vi "Divide Quaternion by Scalar.vi"(1 "y":dbl, 2 "quaternion":T1) -> (0 "quotient":T1)   [LabVIEW 2017, in "NI_Kinematics.lvlib"]
doc: "Computes the <B>quotient</B> of two quaternions or a quaternion and a scalar number. Wire data to the <B>y</B> input to determine the polymorphic instance to use or manually select the instance."
uses:
  <vilib>/robotics/Kinematics/NI_Kinematics.lvlib
  <vilib>/robotics/Kinematics/Quaternion.ctl
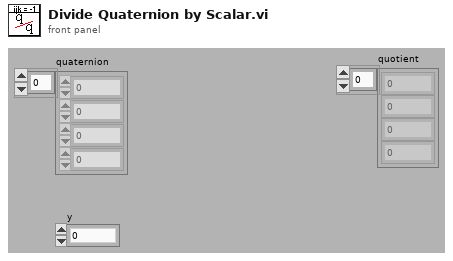
[diagram p1: front panel]
types:
  T1 = typedef "NI_Kinematics.lvlib/Quaternion.ctl" = dbl[]
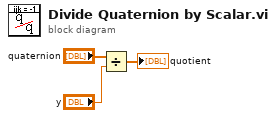
[diagram p0: block diagram]
diagram:
  n1 = Divide(x="quaternion", y="y") -> (x/y=→"quotient":T1)
